vi "GE 5565PIORC.DMA.Scatter-Gather.Commit Linked Block Descriptors.vi"(8 "error in (no error)":errorcluster, 10 "Linked Block Descriptors":T1[](array[typedef]) {"descriptor params"."data ptr (lower)" format="%.0x"; "descriptor params"."data ptr (upper)" format="%.0x"; "descriptor params"."data size" format="%.0x"; "descriptor params"."next descriptor ptr" format="%.0x"; "descriptor size" format="%08x"; "descriptor ptr (RFM)" format="%08x"; "descriptor ptr (VISA)" format="%08x"}, 11 "GE 5565PIORC in":refnum<class "GE 5565PIORC.lvclass">) -> (0 "error out":errorcluster, 3 "GE 5565PIORC out":refnum<class "GE 5565PIORC.lvclass">)   [LabVIEW 2017, in "GE 5565PIORC.lvclass"]
doc: "Commits the provided <B>Linked Block Descriptors</B> to PCI memory."
uses:
  GE 5565PIORC.lvclass
  Typedefs/GE 5565PIORC.Typedef.DMA Block Descriptor.ctl
  Typedefs/GE 5565PIORC.Typedef.DMA Block Descriptor Params.ctl
  GE 5565PIORC.lvclass/GE 5565PIORC.ctl
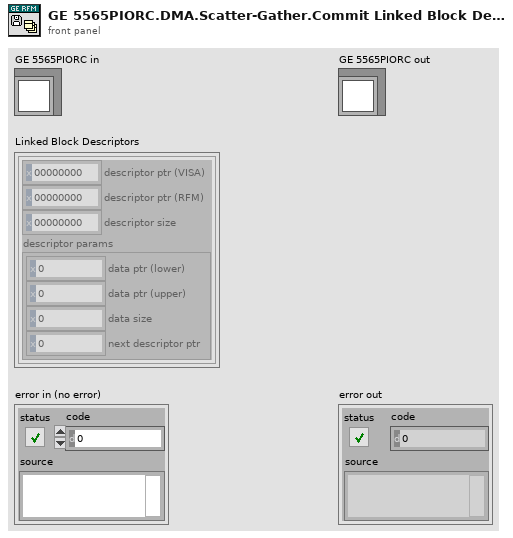
[diagram p1: front panel]
types:
  T1 = typedef "GE 5565PIORC.lvclass/GE 5565PIORC.Typedef.DMA Block Descriptor.ctl" = cluster{"descriptor ptr (VISA)":u32, "descriptor ptr (RFM)":u32, "descriptor size":u32, "descriptor params":T2}
  T2 = typedef "GE 5565PIORC.lvclass/GE 5565PIORC.Typedef.DMA Block Descriptor Params.ctl" = cluster{"data ptr (lower)":u32, "data ptr (upper)":u32, "data size":u32, "next descriptor ptr":u32}
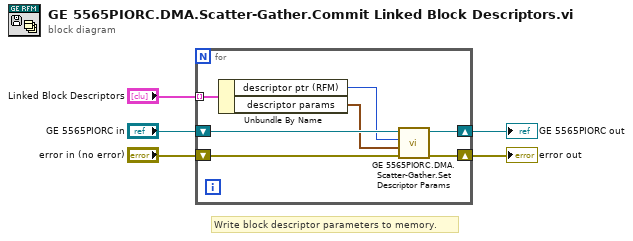
[diagram p0: block diagram]
diagram:
  # "Write block descriptor parameters to memory."
  n1 = for {
    tunnel: "Linked Block Descriptors" -> [w12] mode=indexing
    shift-right: [w9] -> w3
    shift-left: "error in (no error)" -> [w11]
    shift-right: [w8] -> w1
    shift-left: "GE 5565PIORC in" -> [w10]
    n2 = Unbundle By Name(w12) -> ("descriptor ptr (RFM)"=w6:u32, "descriptor params"=w7:T2)
    n3 = call "GE 5565PIORC.DMA.Scatter-Gather.Set Descriptor Params.vi"("error in (no error)"=w11, "descriptor params"=w7, "descriptor ptr"=w6, "GE 5565PIORC in"=w10) -> ("error out"=w9:errorcluster, "GE 5565PIORC out"=w8:refnum<class "GE 5565PIORC.lvclass">)  [unwired: 6 in]
  }
  "GE 5565PIORC out" <- w1
  "error out" <- w3
